vi "Init.vi"(8 "error in (no error)":errorcluster, 10 "Node Info":T1) -> (0 "error out":errorcluster, 3 "Node out":refnum<class "Node Config.lvclass">)   [LabVIEW 2020, in "Vecto.lvlib" / "Node Config.lvclass"]
uses:
  Node Config.lvclass
  Node Config.lvclass/Node Config.ctl
  Node Info.ctl
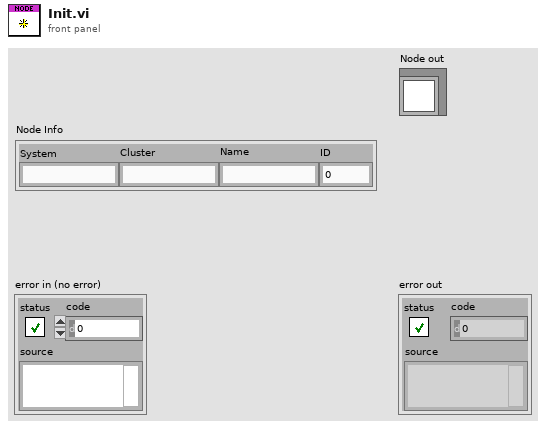
[diagram p1: front panel]
types:
  T1 = typedef "Vecto.lvlib/Node Config.lvclass/Node Info.ctl" = cluster{"System":string, "Cluster":string, "Name":string, "ID":u32}
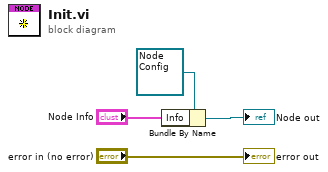
[diagram p0: block diagram]
diagram:
  n1 = Bundle By Name(cluster=refnum<class "Node Config.lvclass"> refnum ("Node in"), "Info"="Node Info") -> (→"Node out":refnum<class "Node Config.lvclass">)
  "error out" <- "error in (no error)"
